vi "Phasics phase array to image.vi"(6 "Phase in":sgl[][](array[numeric]), 8 "error in (no error)":errorcluster, 11 "Phasics Camera in":refnum<class "Phasics Camera.lvclass">) -> (0 "error out":errorcluster, 3 "Phasics Camera out":refnum<class "Phasics Camera.lvclass">)   [LabVIEW 2013, in "Phasics Camera.lvclass"]
uses:
  Phasics Camera.lvclass
  Phasics Camera.lvclass/Phasics Camera.ctl
  CompressAndUpdate(IMAQ Image).vi
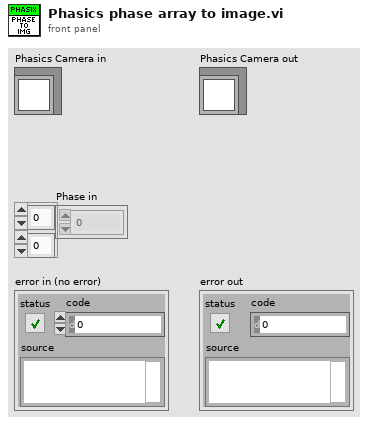
[diagram p1: front panel]
types:
  T1 = typedef "IMAQ Image.ctl" = refnum<image>
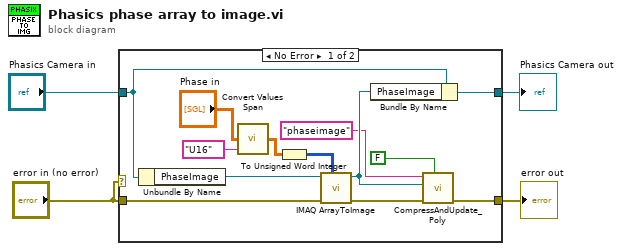
[diagram p0: block diagram]
diagram:
  n1 = case shown="No Error" "error in (no error)" {
    tunnel: [w17 w18] -> w4
    tunnel: [w15 w19] -> w3
    tunnel: "error in (no error)" -> [w8 w19]
    tunnel: "Phasics Camera in" -> [w6 w18]
    frame No Error {
      n2 = Unbundle By Name(w6) -> ("PhaseImage"=w5:T1)
      n3 = call "Convert Values Span.vi"("Input Array"="Phase in", "Data type"="U16") -> ("Output Array"=w10:sgl[][])  [unwired: 5 in]
      n4 = To Unsigned Word Integer(number=w10) -> (unsigned 16bit integer=w14:u16[][])
      n5 = call "IMAQ ArrayToImage"("Image Pixels (U16)"=w14, "error in (no error)"=w8, "Image"=w5) -> ("error out"=w13:errorcluster, "Image Out"=w16:T1)  [unwired: 7 in]
      n6 = Bundle By Name(cluster=w6, "PhaseImage"=w16) -> (w17:refnum<class "Phasics Camera.lvclass">)
      n7 = call-poly "CompressAndUpdate_Poly.vi"("force CVT update (false)"=FALSE, "error in"=w13, "IMAQ Image"=w16, "command or variable name"="phaseimage") -> ("error out"=w15:errorcluster)  [unwired: 7 in]
    }
    frame Error {
    }
  }
  "Phasics Camera out" <- w4
  "error out" <- w3
